vi "poly_data_queue_ctrl.vi"(5 "skip? (F)":bool, 6 "initial queue element (not a refnum)":refnum<vi>, 7 "initialize":bool, 8 "error in":errorcluster caption="Error in (no error)", 9 "queue length (100)":i32=100, 10 "input data point":refnum<vi>) -> (0 "error out":errorcluster, 1 "eliminated element":refnum<vi>, 2 "queue":refnum<vi>[](array[refnum]), 4 "current length":i32)   [LabVIEW 2015]
uses:
  poly_average_tools_eco_plus.vi
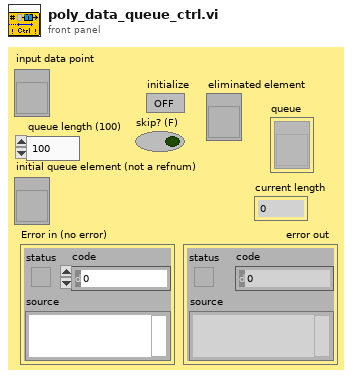
[diagram p1: front panel]
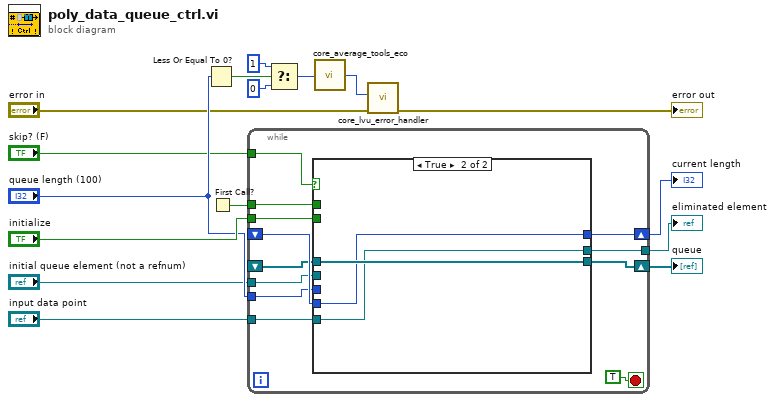
[diagram p0: block diagram]
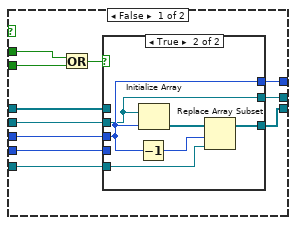
[diagram p2: hidden frame]
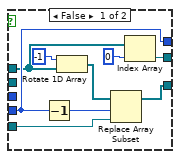
[diagram p3: hidden frame]
diagram:
  n1 = Less Or Equal To 0?(x="queue length (100)") -> (x <= 0?=w12:bool)
  n2 = First Call?() -> (First Call?: T/F=w13:bool)
  n3 = while {
    tunnel: w13 -> [w23]
    shift-left: _ -> [w26]
    shift-right: [w27] -> w16
    shift-left: _ -> [w25]
    shift-right: [w28] -> w5
    tunnel: "initialize" -> [w22]
    tunnel: "input data point" -> [w21]
    tunnel: "initial queue element (not a refnum)" -> [w20]
    tunnel: "queue length (100)" -> [w19]
    tunnel: [w18] -> w4
    tunnel: "skip? (F)" -> [w17]
    stop <- TRUE stop-if-true
    n4 = case shown="True" w17 {
      tunnel: [w39 w57] -> w28
      tunnel: [w38 w55] -> w27
      tunnel: w26 -> [w37 w55]
      tunnel: w25 -> [w36 w57]
      tunnel: w23 -> [w35 _]
      tunnel: w22 -> [w33 _]
      tunnel: w21 -> [w32 w56]
      tunnel: w20 -> [w31 _]
      tunnel: w19 -> [w30 _]
      tunnel: [w29 w56] -> w18
      frame False {
        n5 = Or(x=w35, y=w33) -> (x .or. y?=w34:bool)
        n6 = case shown="True" w34 {
          tunnel: [w45 w50] -> w39
          tunnel: [w46 w53] -> w38
          tunnel: w37 -> [w46 _]
          tunnel: w36 -> [w42 _]
          tunnel: w32 -> [w47 w51]
          tunnel: w31 -> [_ w49]
          tunnel: w30 -> [_ w53]
          tunnel: [w40 w49] -> w29
          frame False {
            n7 = Decrement(x=w46) -> (x-1=w44:i32)
            n8 = Rotate 1D Array(1:w42, 2:i16 -1 ("n")) -> (0:w43:refnum<vi>[])
            n9 = Replace Array Subset(array=w43, new element=w47, index=w44) -> (w45:refnum<vi>[])
            n10 = Index Array(array=w42, index=0 ("Index")) -> (element=w40:refnum<vi>)
          }
          frame True {
            n11 = Decrement(x=w53) -> (x-1=w54:i32)
            n12 = Initialize Array(w49, w53) -> (w52:refnum<vi>[])
            n13 = Replace Array Subset(array=w52, new element=w51, index=w54) -> (w50:refnum<vi>[])
          }
        }
      }
      frame True {
      }
    }
  }
  "current length" <- w16
  "queue" <- w5
  "eliminated element" <- w4
  n14 = Select(t=1, s=w12, f=0) -> (s? t:f=w2:i32)
  n15 = call-poly "core_average_tools_eco.vi"("code (w/out eco)"=w2) -> ("code (+ eco)"=w1:i32)  [unwired: 4 in]
  n16 = call "core_lvu_error_handler.vi"("error in (no error)"="error in", "code (0 = no error)"=w1) -> ("error out"=→"error out":errorcluster)  [unwired: 8 in, 1 out]
